vi "SAW_Jeremy2019.vi"() -> ()   [LabVIEW 2019]
panel:
  out "S11":dbl[][](graph)
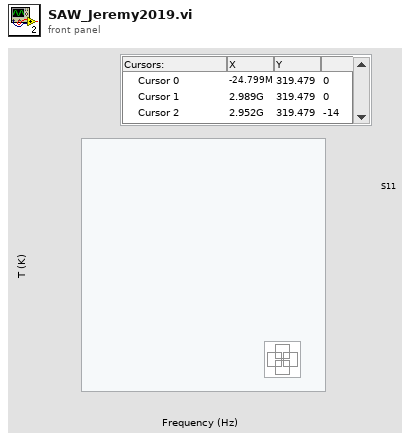
[diagram p1: front panel]
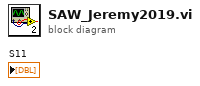
[diagram p0: block diagram]
diagram:
